vi "xyz AE.vi"() -> ()   [LabVIEW 2020]
uses:
  typedef_stage_control.ctl
panel:
  out "Z Position":dbl
  out "Y Position":dbl
  out "X Position":dbl
  in  "Cluster":T1={"Up"=FALSE, "Left"=FALSE, "Right"=FALSE, "Down"=FALSE, "Focus Down"=FALSE, "Focus Up"=FALSE, "X Step Size(um)"=6.860690000000502, "Z step size (um)"=100.0, "Y Step Size(um)"=100.0, "X Position"=0.0, "Y Position"=0.0, "Z Position"=0.0, "Enable x-axis"=TRUE, "Enable y-axis"=TRUE, "Enable z-axis"=TRUE}
  out "Connected":bool=TRUE
  out "GetFirmwareVersion":string="3.03\r"
  in  "SPIIPLUSCOM660Lib.IAsyncChannel":refnum<k7>
  out "Error out":errorcluster
  in  "stop":bool
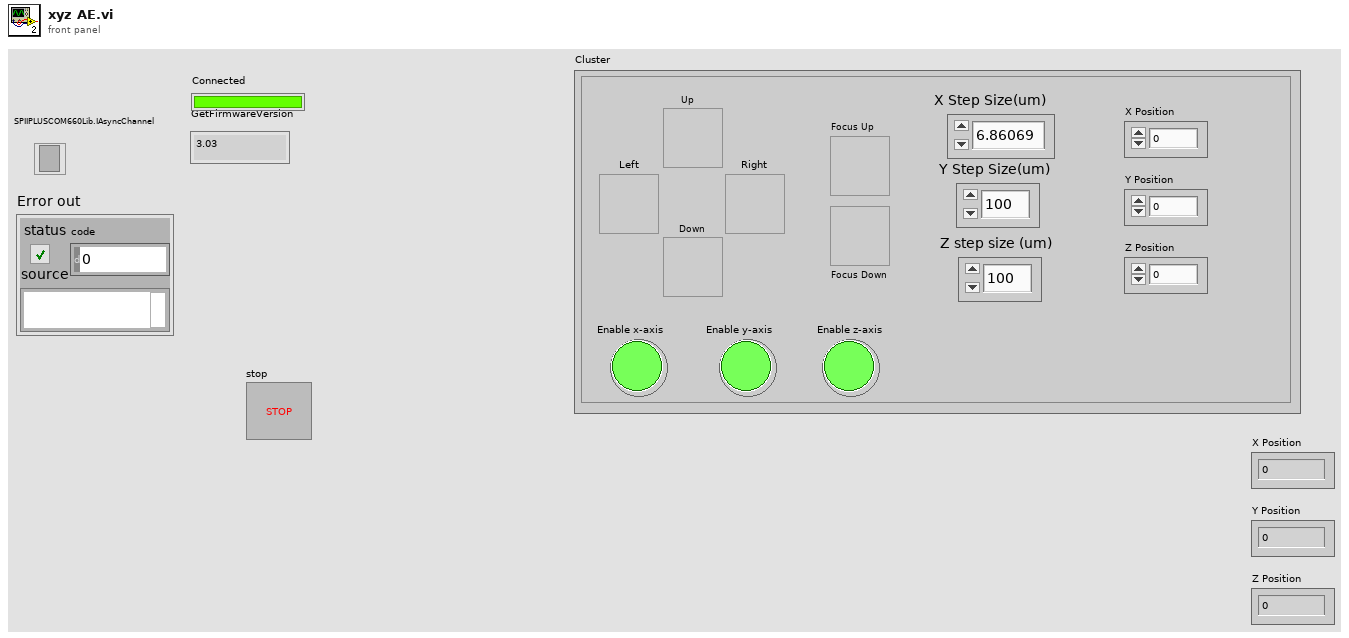
[diagram p1: front panel]
types:
  T1 = typedef "typedef_stage_control.ctl" = cluster{"Up":bool, "Left":bool, "Right":bool, "Down":bool, "Focus Down":bool, "Focus Up":bool, "X Step Size(um)":dbl, "Z step size (um)":dbl, "Y Step Size(um)":dbl, "X Position":dbl, "Y Position":dbl, "Z Position":dbl, "Enable x-axis":bool, "Enable y-axis":bool, "Enable z-axis":bool}
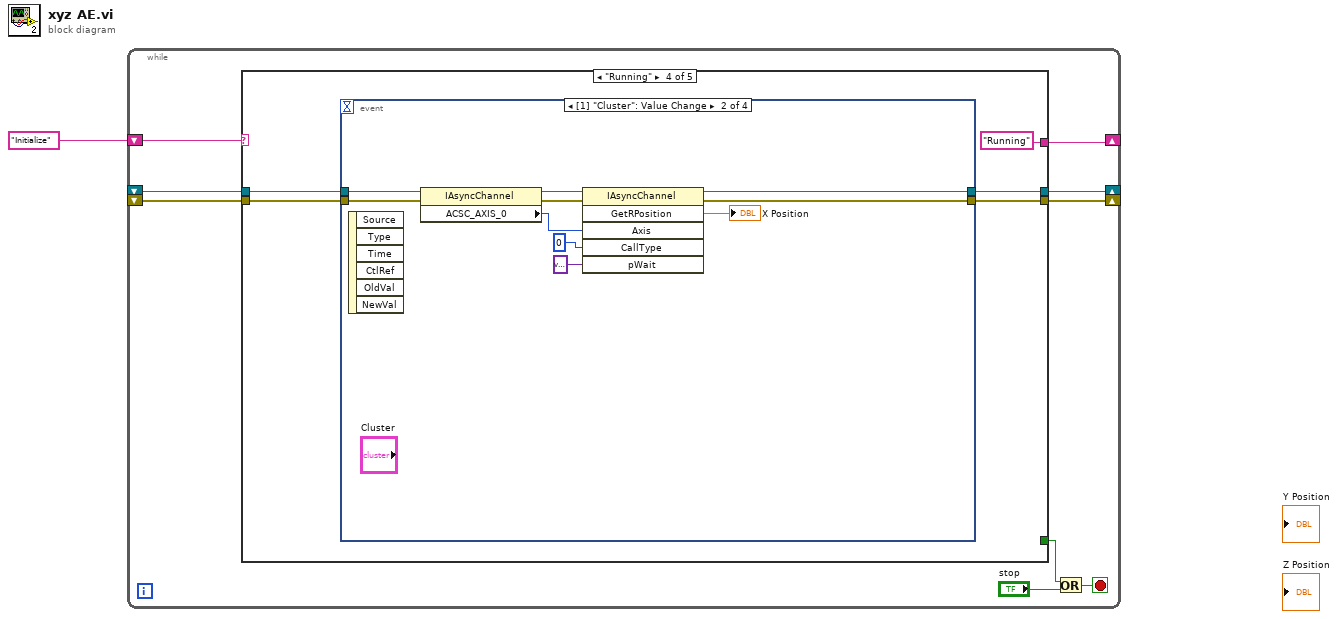
[diagram p0: block diagram]
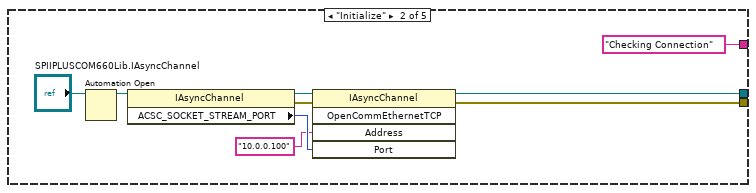
[diagram p3: hidden frame]
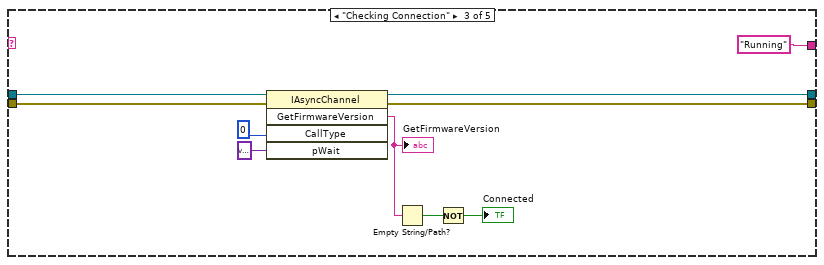
[diagram p4: hidden frame]
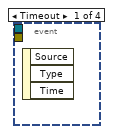
[diagram p5: hidden frame]
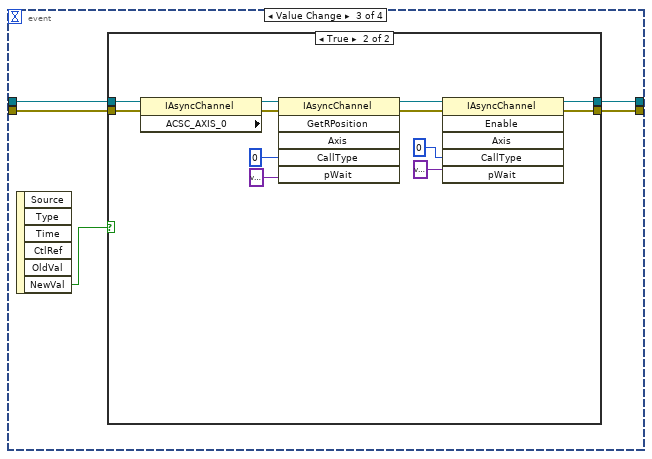
[diagram p6: hidden frame]
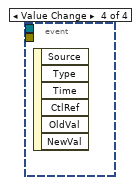
[diagram p8: hidden frame]
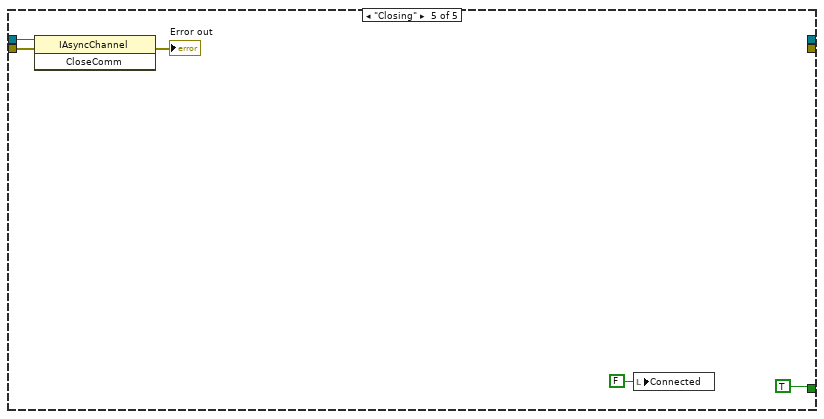
[diagram p9: hidden frame]
diagram:
  n1 = while {
    shift-right: [w10] -> _
    shift-left: _ -> [w7]
    shift-right: [w9] -> _
    shift-left: _ -> [w8]
    shift-right: [w5] -> _
    shift-left: "Initialize" -> [w6]
    stop <- w4 stop-if-true
    n2 = case shown="\"Running\"" w6 {
      tunnel: [_ w13 w24 w31 _] -> w10
      tunnel: [_ w12 w23 w30 _] -> w9
      tunnel: w8 -> [_ _ w22 w33 w63]
      tunnel: w7 -> [_ _ w21 w34 w64]
      tunnel: [_ "Checking Connection" "Running" "Running" _] -> w5
      tunnel: [_ _ _ _ TRUE] -> w2
      frame "False", Default {
      }
      frame "Initialize" {
        n3 = Automation Open(Automation Refnum="SPIIPLUSCOM660Lib.IAsyncChannel") -> (Automation Refnum=w19:refnum<k7>)  [unwired: 3 in, 1 out]
        n4 = property class="IAsyncChannel"(reference=w19) -> (reference out=w18:refnum<k7>, error out=w14:errorcluster, "ACSC_SOCKET_STREAM_PORT"=w16:i32)  [unwired: 1 in]
        n5 = invoke class="IAsyncChannel" method="OpenCommEthernetTCP"(reference=w18, error in=w14, "Address"="10.0.0.100", "Port"=w16) -> (reference out=w13:refnum<k7>, error out=w12:errorcluster)  [unwired: 1 in, 3 out]
      }
      frame "Checking Connection" {
        n6 = invoke class="IAsyncChannel" method="GetFirmwareVersion"(reference=w21, error in=w22, "CallType"=u64 0, "pWait"=variant) -> (reference out=w24:refnum<k7>, error out=w23:errorcluster, "GetFirmwareVersion"=w27:string)  [unwired: 1 in, 2 out]
        "GetFirmwareVersion" <- w27
        n7 = Empty String/Path?(string/path=w27) -> (empty?=w26:bool)
        n8 = Not(x=w26) -> (.not. x?=→"Connected":bool)
      }
      frame "Running" {
        n9 = event shown="[1] \"Cluster\": Value Change" {
          selector: _ -> [_ _ _ _]
          dyn-events: _ -> [_ _ _ _]
          timeout: _ -> [_ _ _ _]
          tunnel: w34 -> [_ w39 w46 _]
          tunnel: w33 -> [_ w38 w45 _]
          tunnel: [_ w37 w48 _] -> w31
          tunnel: [_ w36 w47 _] -> w30
          event Timeout {
            n10 = event-data() -> ()  [unwired: 1 in, 3 out]
          }
          event Value Change {
            n11 = event-data() -> ()  [unwired: 1 in, 6 out]
            n12 = property class="IAsyncChannel"(reference=w39, error in=w38) -> (reference out=w44:refnum<k7>, error out=w43:errorcluster, "ACSC_AXIS_0"=w42:i32)
            n13 = invoke class="IAsyncChannel" method="GetRPosition"(reference=w44, error in=w43, "Axis"=w42, "CallType"=u64 0, "pWait"=variant) -> (reference out=w37:refnum<k7>, error out=w36:errorcluster, "GetRPosition"=→"X Position":dbl)  [unwired: 1 in, 3 out]
          }
          event Value Change {
            n14 = event-data() -> ("NewVal"=w49:bool)  [unwired: 1 in, 5 out]
            n15 = case shown="True" w49 {
              tunnel: [_ w53] -> w48
              tunnel: [_ w52] -> w47
              tunnel: w46 -> [_ w51]
              tunnel: w45 -> [_ w50]
              frame False {
              }
              frame True {
                n16 = property class="IAsyncChannel" props=["ACSC_AXIS_0"](reference=w51, error in=w50) -> (reference out=w57:refnum<k7>, error out=w56:errorcluster)  [unwired: 1 out]
                n17 = invoke class="IAsyncChannel" method="GetRPosition"(reference=w57, error in=w56, "CallType"=u64 0, "pWait"=variant) -> (reference out=w58:refnum<k7>, error out=w59:errorcluster)  [unwired: 2 in, 4 out]
                n18 = invoke class="IAsyncChannel" method="Enable"(reference=w58, error in=w59, "CallType"=u64 0, "pWait"=variant) -> (reference out=w53:refnum<k7>, error out=w52:errorcluster)  [unwired: 2 in, 4 out]
              }
            }
          }
          event Value Change {
            n19 = event-data() -> ()  [unwired: 1 in, 6 out]
          }
        }
      }
      frame "Closing" {
        n20 = invoke class="IAsyncChannel" method="CloseComm"(reference=w64, error in=w63) -> (error out=→"Error out":errorcluster)  [unwired: 1 in, 2 out]
        n21 = local write "Connected"(FALSE ("Connected")) -> ()
      }
    }
    n22 = Or(x=w2, y="stop") -> (x .or. y?=w4:bool)
  }
